vi "Launcher - SerialComm.vi"() -> ()   [LabVIEW 2014]
uses:
  Workers/SerialComm/SerialComm.lvclass
panel:
  out "error out":errorcluster
  in  "error in":errorcluster
  # "Entry point"
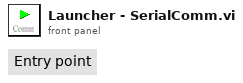
[diagram p1: front panel]
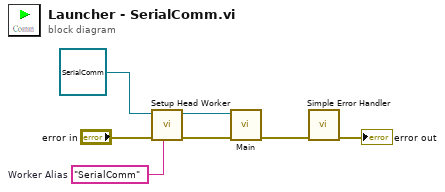
[diagram p0: block diagram]
diagram:
  w1 = "SerialComm"  # Worker Alias
  n1 = call-dynamic "Setup Head Worker.vi"("Worker Alias"=w1, "error in"="error in", "Worker"=refnum<class "SerialComm.lvclass"> refnum ("Worker User Object")) -> ("error out"=w7:errorcluster, "Worker out"=w4:refnum<class "SerialComm.lvclass">)  [unwired: 7 in]
  n2 = call-dynamic "Main.vi"("error in"=w7, "SerialComm in"=w4) -> ("error out"=w5:errorcluster)  [unwired: 8 in, 1 out]
  n3 = call <vilib>:"Simple Error Handler.vi"("error in (no error)"=w5) -> ("error out"=→"error out":errorcluster)  [unwired: 4 in, 4 out]
